vi "array to x axis set.vi"(7 "smooth n":dbl=1.0, 11 "1d Data":dbl[](array[numeric])) -> (2 "offset":dbl, 3 "multiplier":dbl)   [LabVIEW 2024]
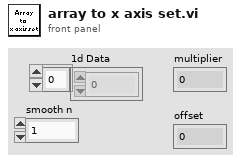
[diagram p1: front panel]
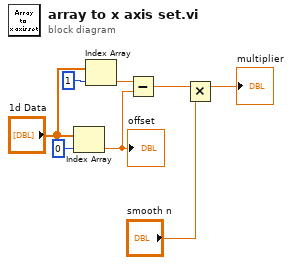
[diagram p0: block diagram]
diagram:
  n1 = Index Array(array="1d Data", index=0) -> (element=w8:dbl)
  "offset" <- w8
  n2 = Index Array(array="1d Data", index=1 ("index (row)")) -> (element=w5:dbl)
  n3 = Subtract(x=w5, y=w8) -> (x-y=w7:dbl)
  n4 = Multiply(x=w7, y="smooth n") -> (x*y=→"multiplier":dbl)
